vi "init_delay_generator.vi"(5 "polarity":string[](array[string])=["1", "0", "1", "0", "1"], 6 "power level":string="4.0", 7 "VISA resource name":refnum<visa-resource-name>="TRIG") -> (0 "error out":errorcluster, 3 "VISA resource name out":refnum<visa-resource-name>)   [LabVIEW 2011]
doc: "Initializes the delay generator to the defaults settings, leaves the delay data untouched."
panel:
  # "nozzle"
  # "power amp"
  # "AWG"
  # "SWITCH polarity"
  # "OSC"
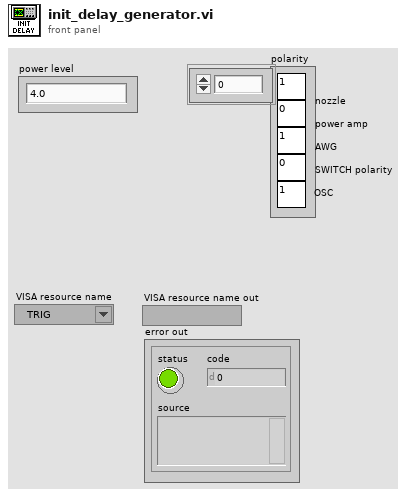
[diagram p1: front panel]
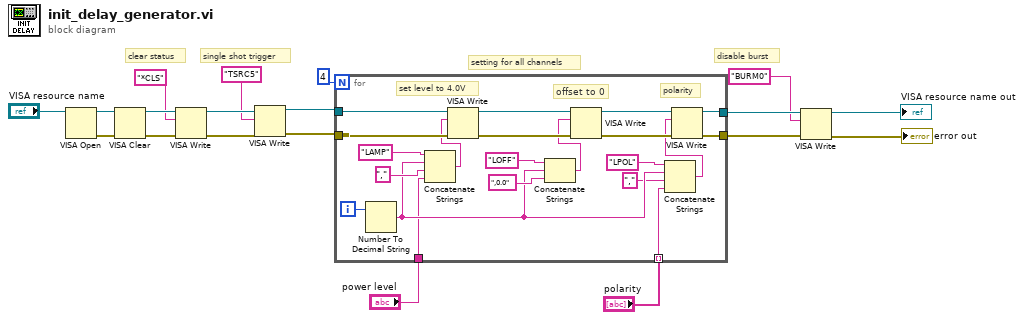
[diagram p0: block diagram]
diagram:
  # "setting for all channels"
  # "disable burst"
  # "clear status"
  # "single shot trigger"
  n1 = VISA Open(VISA resource name="VISA resource name") -> (VISA resource name=w18:refnum<visa-resource-name>, error out=w19:errorcluster)  [unwired: 4 in]
  n2 = VISA Clear(VISA resource name=w18, error in (no error)=w19) -> (VISA resource name out=w17:refnum<visa-resource-name>, error out=w16:errorcluster)
  n3 = VISA Write(VISA resource name=w17, write buffer="*CLS" ("Query 2"), error in (no error)=w16) -> (VISA resource name out=w13:refnum<visa-resource-name>, error out=w12:errorcluster)  [unwired: 1 out]
  n4 = VISA Write(VISA resource name=w13, write buffer="TSRC5" ("Query 2"), error in (no error)=w12) -> (VISA resource name out=w7:refnum<visa-resource-name>, error out=w5:errorcluster)  [unwired: 1 out]
  n5 = for {
    N: 4 -> [_]
    tunnel: w7 -> [w39]
    tunnel: [w26] -> w6
    tunnel: w5 -> [w38]
    tunnel: [w28] -> w4
    tunnel: "polarity" -> [w22] mode=indexing
    tunnel: "power level" -> [w20]
    i -> [w36]
    # "polarity"
    # "offset to 0"
    # "set level to 4.0V"
    n6 = Number To Decimal String(number=w36) -> (decimal integer string=w24:string)  [unwired: 1 in]
    n7 = Concatenate Strings("LAMP" ("Query 2"), w24, "," ("Query 2"), w20) -> (w34:string)
    n8 = VISA Write(VISA resource name=w39, write buffer=w34, error in (no error)=w38) -> (VISA resource name out=w30:refnum<visa-resource-name>, error out=w37:errorcluster)  [unwired: 1 out]
    n9 = Concatenate Strings("LOFF" ("Query 2"), w24, ",0.0" ("Query 2")) -> (w29:string)
    n10 = VISA Write(VISA resource name=w30, write buffer=w29, error in (no error)=w37) -> (VISA resource name out=w27:refnum<visa-resource-name>, error out=w31:errorcluster)  [unwired: 1 out]
    n11 = Concatenate Strings("LPOL" ("Query 2"), w24, "," ("string"), w22) -> (w23:string)
    n12 = VISA Write(VISA resource name=w27, write buffer=w23, error in (no error)=w31) -> (VISA resource name out=w26:refnum<visa-resource-name>, error out=w28:errorcluster)  [unwired: 1 out]
  }
  n13 = VISA Write(VISA resource name=w6, write buffer="BURM0", error in (no error)=w4) -> (VISA resource name out=→"VISA resource name out":refnum<visa-resource-name>, error out=→"error out":errorcluster)  [unwired: 1 out]
